vi "Edit illegal filenames.vi"() -> ()   [LabVIEW 2020]
panel:
  out "Target path":path
  out "Source path":path
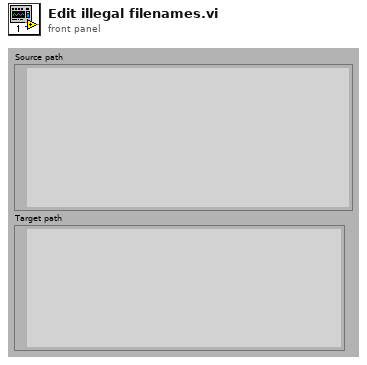
[diagram p1: front panel]
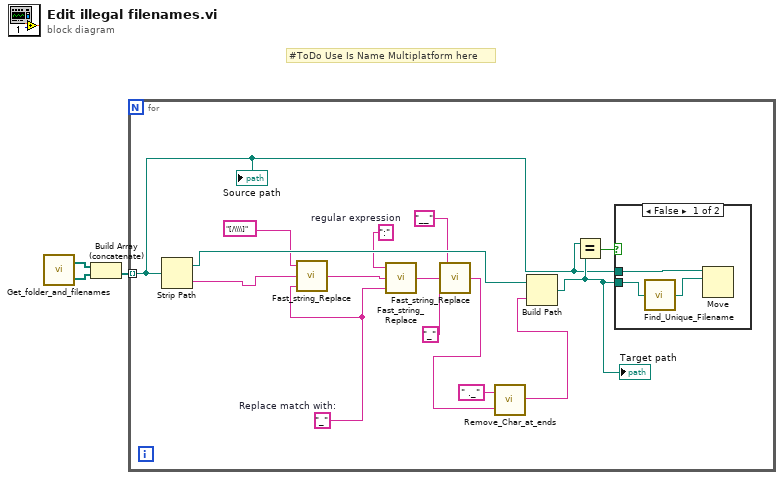
[diagram p0: block diagram]
diagram:
  # "#ToDo Use Is Name Multiplatform here"
  n1 = call "Get_folder_and_filenames.vi"() -> ("Folders"=w3:path[], "Files"=w2:path[])  [unwired: 1 in]
  n2 = Build Array (concatenate)(w3, w2) -> (w1:path[])
  n3 = for {
    tunnel: w1 -> [w7] mode=indexing
    w11 = "_"  # Replace match with:
    w15 = ":"  # regular expression
    n4 = Strip Path(path=w7) -> (stripped path=w17:path, name=w18:string)
    n5 = call "Fast_string_Replace.vi"("Replace match with:"=w11, "Input String"=w18, "regular expression"="[/\\\\]") -> ("Output String"=w16:string)  [unwired: 1 in, 1 out]
    n6 = call "Fast_string_Replace.vi"("Replace match with:"=w11, "Input String"=w16, "regular expression"=w15) -> ("Output String"=w12:string)  [unwired: 1 in, 1 out]
    n7 = call "Fast_string_Replace.vi"("Replace match with:"="_", "Input String"=w12, "regular expression"="__") -> ("Output String"=w5:string)  [unwired: 1 in, 1 out]
    n8 = call "Remove_Char_at_ends.vi"("String in"=w5, "Characters to remove"=" ._" ("Character to remove")) -> ("String out"=w4:string)
    n9 = Build Path(base path=w17, name or relative path=w4) -> (appended path=w9:path)
    "Target path" <- w9
    n10 = Equal?(x=w7, y=w9) -> (x = y?=w8:bool)
    n11 = case shown="False" w8 {
      tunnel: w7 -> [w21 _]
      tunnel: w9 -> [w20 _]
      frame False {
        n12 = call "Find_Unique_Filename.vi"("Path In"=w20) -> ("Unique Path Out"=w19:path)  [unwired: 2 in]
        n13 = Move(source path=w21, 10:w19) -> ()  [unwired: 3 in, 3 out]
      }
      frame True {
      }
    }
    "Source path" <- w7
  }
